vi "fo_SelectWorklistItem.vi"(8 "error in (no error)":errorcluster) -> (0 "error out":errorcluster, 2 "items":string[](array[string]), 3 "tags":string[](array[string]))   [LabVIEW 2013, in "main.lvlib"]
uses:
  main.lvlib
  C:/Users/Simon/SkyDrive/LabView/2013/DM2020/bin/Dicom.dll
  bin/Dicom.dll
panel:
  in  "DicomDatasets":refnum<k24>
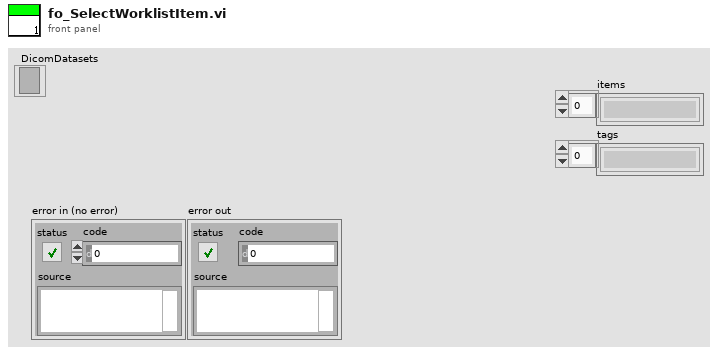
[diagram p1: front panel]
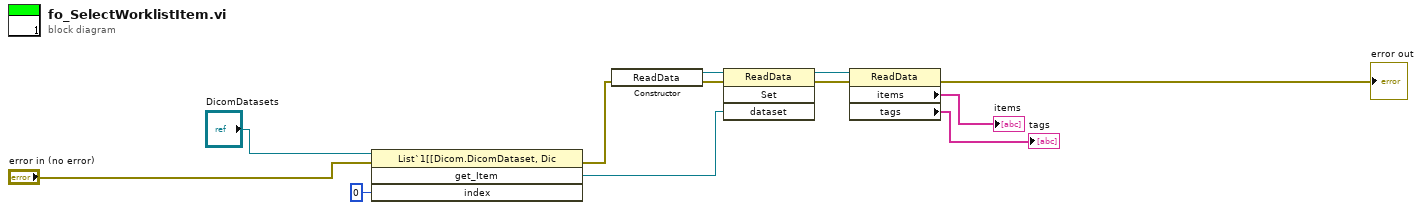
[diagram p0: block diagram]
diagram:
  n1 = invoke class="List`1[[Dicom.DicomDataset, Dic" method="get_Item"(reference="DicomDatasets", error in="error in (no error)", "index"=0) -> (error out=w8:errorcluster, "get_Item"=w10:refnum<k24>)  [unwired: 1 in, 2 out]
  n2 = constructor class="ReadData"(error in=w8) -> (reference out=w12:refnum<k24>, error out=w9:errorcluster)  [unwired: 2 in, 1 out]
  n3 = invoke class="ReadData" method="Set"(reference=w12, error in=w9, "dataset"=w10) -> (reference out=w2:refnum<k24>, error out=w1:errorcluster)  [unwired: 1 in, 2 out]
  n4 = property class="ReadData"(reference=w2, error in=w1) -> (error out=→"error out":errorcluster, "items"=→"items":string[], "tags"=→"tags":string[])  [unwired: 1 out]
